vi "errorDisp.vi"(9 "error path index in":i32, 10 "error?":bool, 11 "string check in":string) -> (1 "string check":string, 2 "path index":string, 3 "true":bool)   [LabVIEW 2015, in "Zen Analytics.lvclass"]
uses:
  Zen Analytics.lvclass
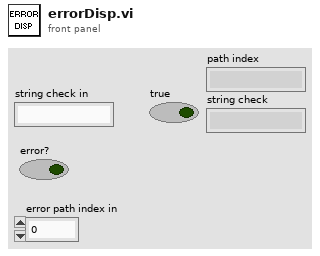
[diagram p1: front panel]
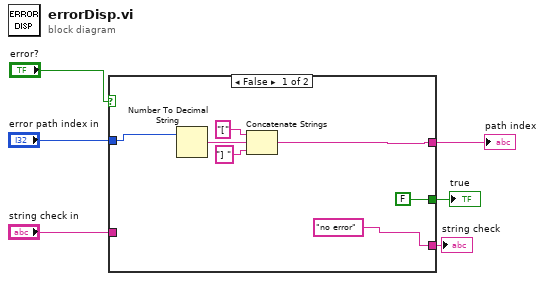
[diagram p0: block diagram]
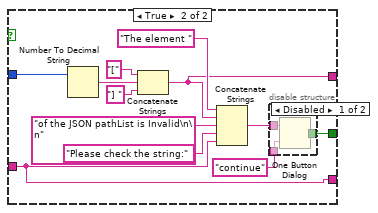
[diagram p2: hidden frame]
diagram:
  n1 = case shown="False" "error?" {
    tunnel: "error path index in" -> [w9 w25]
    tunnel: [FALSE ("true") w20] -> w4
    tunnel: "string check in" -> [_ w15]
    tunnel: ["no error" ("string check in") w15] -> w1
    tunnel: [w8 w14] -> w2
    frame False {
      n2 = Number To Decimal String(number=w9) -> (decimal integer string=w10:string)  [unwired: 1 in]
      n3 = Concatenate Strings("[" ("string"), w10, "] " ("string")) -> (w8:string)
    }
    frame True {
      n4 = Number To Decimal String(number=w25) -> (decimal integer string=w16:string)  [unwired: 1 in]
      n5 = Concatenate Strings("[" ("string"), w16, "] " ("string")) -> (w14:string)
      n6 = Concatenate Strings("The element " ("string"), w14, "of the JSON pathList is Invalid\n\n" ("string"), "Please check the string:" ("string"), w15) -> (w22:string)
      n7 = disable-structure shown="Disabled" {
        disable-tunnel: w22 -> [w28 _]
        disable-tunnel: "continue" ("button name (\"OK\")") -> [w27 _]
        disable-tunnel: [w26 _] -> w20
        frame Disabled {
          n8 = One Button Dialog(message=w28, button name ("OK")=w27) -> (true=w26:bool)
        }
        frame Enabled {
        }
      }
    }
  }
  "true" <- w4
  "path index" <- w2
  "string check" <- w1
